vi "Delacor_lib_QMH_Dequeue Message_hjgkjahfd.vi"(8 "error in":errorcluster, 11 "Message Queue in":refnum<class "test class.lvclass">) -> (0 "error out":errorcluster, 1 "Message Data":variant, 2 "Message":string, 3 "Message Queue out":refnum<class "test class.lvclass">)   [LabVIEW 2018, in "test class.lvclass"]
doc: "This VI pulls messages off the Message Queue.\n____\nDQMH Palette 6.0.0.14\nCopyright (c) 2021, DQMH Consortium"
uses:
  SubVIs/test class.lvclass
  <vilib>/Delacor/Delacor QMH/Libraries/Message Queue_class/Delacor_lib_QMH_Message Queue.lvclass
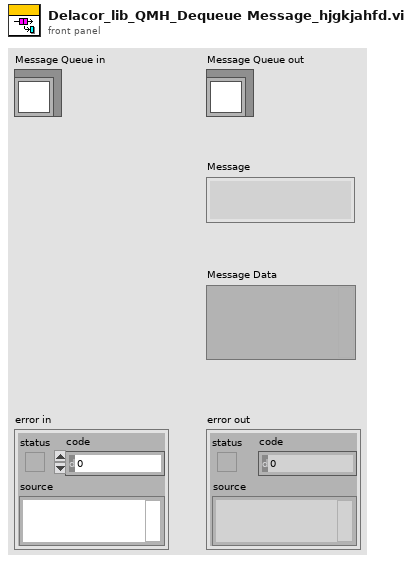
[diagram p1: front panel]
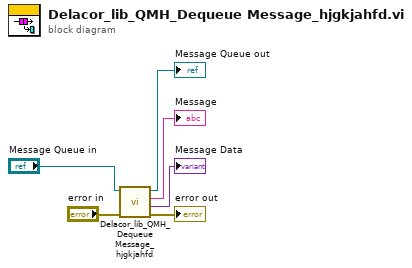
[diagram p0: block diagram]
diagram:
  n1 = call-parent "Delacor_lib_QMH_Dequeue Message_hjgkjahfd.vi"("error in"="error in", "Message Queue in"="Message Queue in") -> ("error out"=→"error out":errorcluster, "Message Data"=→"Message Data":variant, "Message"=→"Message":string, "Message Queue out"=→"Message Queue out":refnum<class "test class.lvclass">)  [unwired: 6 in]
